vi "Update Writable Values.vi"(8 "error in (no error)":errorcluster, 11 "Settings in":refnum<class "Settings.lvclass">) -> (0 "error out":errorcluster, 3 "Settings out":refnum<class "Settings.lvclass">)   [LabVIEW 2017, in "Settings.lvclass"]
uses:
  Settings.lvclass
  Settings.lvclass/Settings.ctl
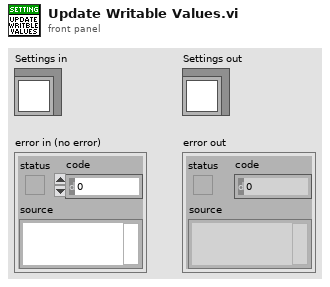
[diagram p1: front panel]
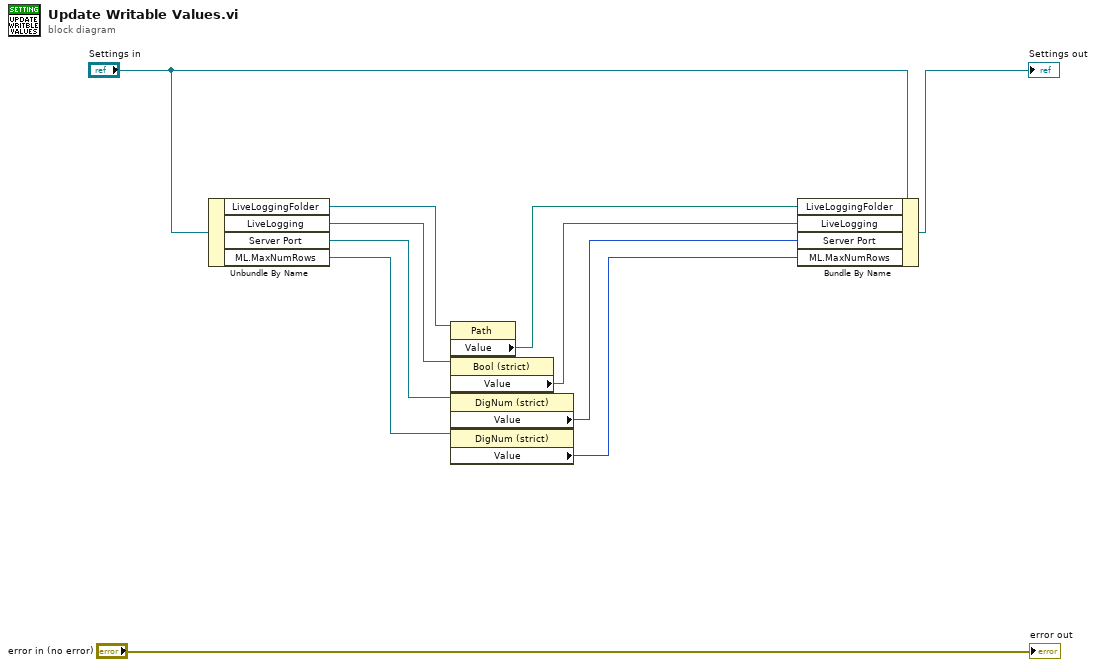
[diagram p0: block diagram]
diagram:
  n1 = Unbundle By Name("Settings in") -> ("LiveLoggingFolder"=w9:refnum<vi>, "LiveLogging"=w8:refnum<vi>, "Server Port"=w10:refnum<vi>, "ML.MaxNumRows"=w7:refnum<vi>)
  n2 = property class="Path"(reference=w9) -> ("Value"=w4:path)  [unwired: 1 in, 2 out]
  n3 = property class="Bool (strict)"(reference=w8) -> ("Value"=w3:bool)  [unwired: 1 in, 2 out]
  n4 = property class="DigNum (strict)"(reference=w10) -> ("Value"=w2:u16)  [unwired: 1 in, 2 out]
  n5 = property class="DigNum (strict)"(reference=w7) -> ("Value"=w1:u16)  [unwired: 1 in, 2 out]
  n6 = Bundle By Name(cluster="Settings in", "LiveLoggingFolder"=w4, "LiveLogging"=w3, "Server Port"=w2, "ML.MaxNumRows"=w1) -> (→"Settings out":refnum<class "Settings.lvclass">)
  "error out" <- "error in (no error)"
